vi "ble_discover_ble_devices.vi"(8 "error in (no error)":errorcluster, 9 "LED ref":refnum<vi>, 10 "Scan Duration (10000ms)":u32=10000, 11 "COM Bluegiga in":refnum<visa-resource-name>) -> (0 "error out":errorcluster, 2 "Devices":string[][](array[string]), 3 "COM Bluegiga out":refnum<visa-resource-name>)   [LabVIEW 2017]
uses:
  type_def/gap_discover_mode.ctl
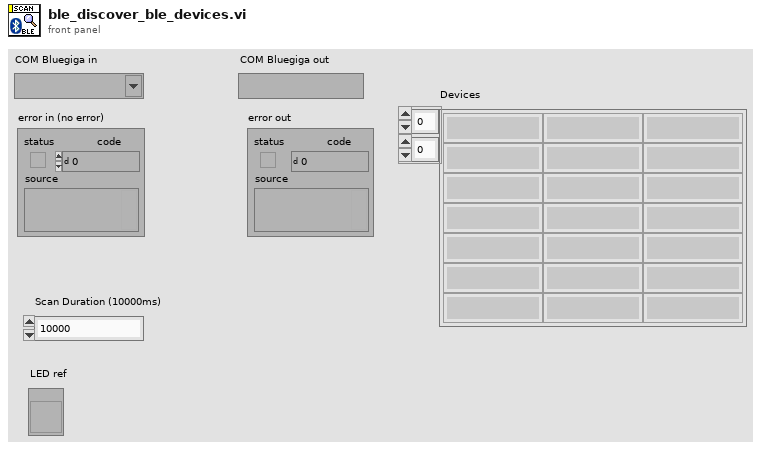
[diagram p1: front panel]
types:
  T1 = typedef "gap_discover_mode.ctl" = u8
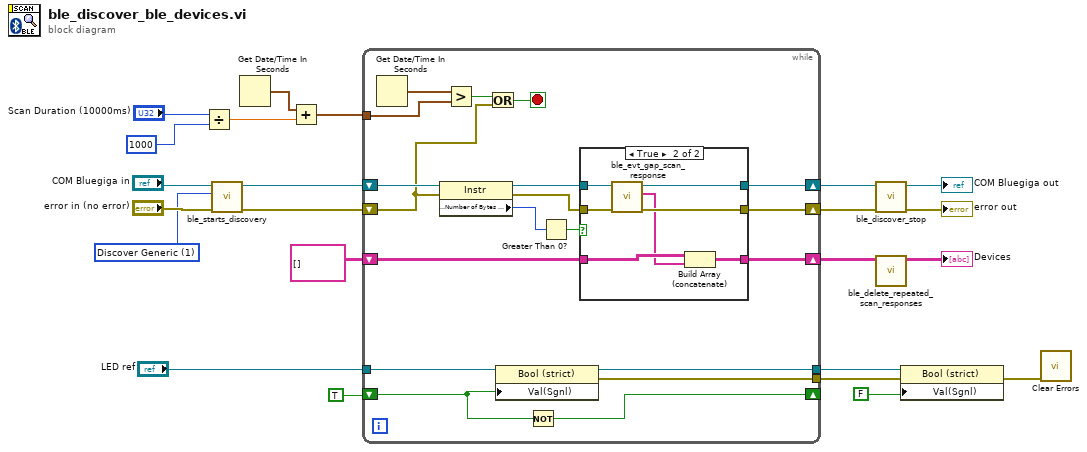
[diagram p0: block diagram]
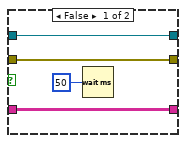
[diagram p2: hidden frame]
diagram:
  w11 = T1 1 items=["Discover Limited", "Discover Generic", "Discover Observation"] ("GAP Discover Mode (Generic)")
  n1 = Divide(x="Scan Duration (10000ms)", y=u32 1000) -> (x/y=w6:dbl)
  n2 = call "ble_starts_discovery.vi"("error in (no error)"="error in (no error)", "GAP Discover Mode (Generic)"=w11, "COM Bluegiga in"="COM Bluegiga in") -> ("error out"=w16:errorcluster, "COM Bluegiga out"=w17:refnum<visa-resource-name>)  [unwired: 5 in, 2 out]
  n3 = Get Date/Time In Seconds() -> (seconds since 1Jan1904=w19:timestamp)
  n4 = Add(x=w19, y=w6) -> (x+y=w18:timestamp)
  n5 = while {
    tunnel: w18 -> [w41]
    shift-right: [w35] -> w14
    shift-left: w17 -> [w40]
    shift-right: [w34] -> w15
    shift-left: w16 -> [w29]
    shift-right: [w30] -> w9
    shift-left: string[][] [] -> [w31]
    tunnel: [w28] -> w4
    tunnel: "LED ref" -> [w27]
    shift-right: [w25] -> _
    shift-left: TRUE -> [w26]
    tunnel: [w24] -> w3
    stop <- w32 stop-if-true
    n6 = Get Date/Time In Seconds() -> (seconds since 1Jan1904=w42:timestamp)
    n7 = property class="Instr"(reference=w40, error in=w29) -> (reference out=w38:refnum<visa-resource-name>, error out=w37:errorcluster, "Serial Settings:Number of Bytes at Serial Port"=w39:u32)
    n8 = Greater?(x=w42, y=w41) -> (0:w33:bool)
    n9 = Or(x=w33, y=w29) -> (x .or. y?=w32:bool)
    n10 = property class="Bool (strict)"(reference=w27, "Val(Sgnl)"=w26) -> (reference out=w24:refnum<vi>, error out=w28:errorcluster)  [unwired: 1 in]
    n11 = Not(x=w26) -> (.not. x?=w25:bool)
    n12 = Greater Than 0?(x=w39) -> (x > 0?=w36:bool)
    n13 = case shown="True" w36 {
      tunnel: w38 -> [w46 w53]
      tunnel: w37 -> [w45 w50]
      tunnel: [w46 w52] -> w35
      tunnel: [w45 w51] -> w34
      tunnel: w31 -> [w43 w49]
      tunnel: [w43 w47] -> w30
      frame False {
        n14 = Wait (ms)(milliseconds to wait=u32 50) -> ()  [unwired: 1 out]
      }
      frame True {
        n15 = call "ble_evt_gap_scan_response.vi"("error in (no error)"=w50, "COM Bluegiga in"=w53) -> ("error out"=w51:errorcluster, "Scan Response 1 Device"=w48:string[], "COM Bluegiga out"=w52:refnum<visa-resource-name>)  [unwired: 7 in]
        n16 = Build Array (concatenate)(w49, w48) -> (w47:string[][])
      }
    }
  }
  n17 = call "ble_discover_stop.vi"("error in (no error)"=w15, "COM Bluegiga in"=w14) -> ("error out"=→"error out":errorcluster, "COM Bluegiga out"=→"COM Bluegiga out":refnum<visa-resource-name>)  [unwired: 6 in, 2 out]
  n18 = call "ble_delete_repeated_scan_responses.vi"("Scan Responses"=w9) -> ("Unique Scan Responses"=→"Devices":string[][])  [unwired: 10 in]
  n19 = property class="Bool (strict)"(reference=w3, error in=w4, "Val(Sgnl)"=FALSE) -> (error out=w2:errorcluster)  [unwired: 1 out]
  n20 = call <vilib>:"Clear Errors.vi"("error in (no error)"=w2) -> ()  [unwired: 5 in, 2 out]
